vi "Get SMO Port.vi"(8 "error in (no error)":errorcluster, 11 "Instrument.Oxford1820 in":refnum<class "Instrument.Oxford1820.lvclass">) -> (0 "error out":errorcluster, 2 "Port":u16, 3 "Instrument.Oxford1820 out":refnum<class "Instrument.Oxford1820.lvclass">)   [LabVIEW 2016, in "Instrument.Oxford1820.lvclass"]
uses:
  Instrument.Oxford1820.lvclass
  <userlib>/LevyLab/Levylab Instruments/Instrument Types/Cryostat/Instrument.Cryostat.lvclass
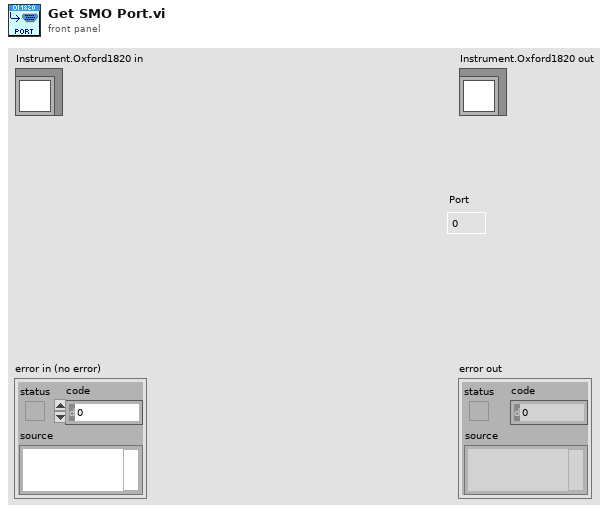
[diagram p1: front panel]
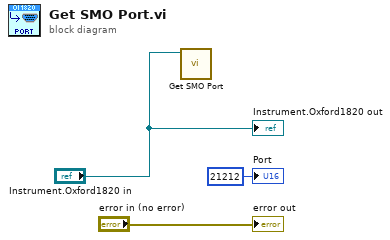
[diagram p0: block diagram]
diagram:
  n1 = call-parent "Get SMO Port.vi"("Instrument in"="Instrument.Oxford1820 in") -> ()  [unwired: 8 in, 3 out]
  "error out" <- "error in (no error)"
  "Instrument.Oxford1820 out" <- "Instrument.Oxford1820 in"
  "Port" <- u16 21212 ("Port")
